vi "PDF_Interface_PDF Protokoll O2 Leaktest.vi"(8 "error in (no error)":errorcluster caption="Fehler (Eingang, kein Fehler)", 11 "Save PDF File Path":path) -> (0 "error out":errorcluster caption="Fehler (Ausgang)")   [LabVIEW 2020, in "O2 Dichtheitstest.lvlib"]
uses:
  O2 Dichtheitstest.lvlib
  Sprachverwaltung/FGV Aktion Tabelle zerlegen.ctl
  Seiten/System Einstellungen V2/Aktioen FGV System Konstanten.ctl
  Aktion FGV O2 Leak.ctl
  PDF_Interface/PDF Protokoll Standard Kopf Optionen.ctl
  <vilib>/Simplicity AI/SAI_PDF_API/Classes/Context/Controls/SAI_PDF_PDF Details.ctl
  PDF_Interface/PDF Interface Helper/PDFContentType.ctl
  PDF_Interface/PDF Interface Helper/PDFTableContentType.ctl
  PDF_Interface/PDF Interface Helper/PDFResults.ctl
  PDF_Interface/PDF Interface Helper/PDFResultPictures.ctl
  PDF_Interface/PDF Interface Helper/PDFCommentPosition.ctl
  PDF_Interface/PDF Interface Helper/PDFPageBreak.ctl
  PDF_Interface/PDF Interface Helper/PDFTablePictures.ctl
  PDF_Interface/PDF Interface Helper/PDFBemerkung.ctl
  <vilib>/Simplicity AI/SAI_PDF_API/Classes/Context/Controls/SAI_PDF_Text Align.ctl
  <vilib>/Simplicity AI/SAI_PDF_API/Classes/Context/Controls/SAI_PDF_Font.ctl
  <vilib>/Simplicity AI/SAI_PDF_API/Classes/Context/Controls/SAI_PDF_Font Encoding.ctl
  Allgemein/allgemeine Sub-VIs.lvlib
  Seiten/System Einstellungen V2/System Einstellungen V2.lvlib
  Sprachverwaltung/Sprachverwaltung.lvlib
  PDF_Interface/PDF Interface.lvlib
  <vilib>/Simplicity AI/SAI_PDF_API/Classes/Context/Context.lvclass
  PDF_Interface/PDF Interface Helper/PDF Interface Helper.lvlib
  Linearisierung V2/Protokoll/Protokoll.lvlib
panel:
  out "Grenzwert Messgasdruck:":string
  out "Messgasdruck:":string
  out "Grenzwert O2:":string
  out "Bestanden":bool caption="Boolesch"
  out "Nullgas Messwert:":string
  out "Datenerfassungszeit:":string
  out "Nullgas Aufschaltzeit:":string
  out "Analysator:":string
  out "Aufschaltpunkt:":string
  out "Endzeit:":string
  out "Startzeit:":string
  out "Ser.Nr.:":string caption="Serien Nummer:"
  out "Messgerät:":string
  # "O2 Leaktest"
  # "s"
  # "s"
  # "kPa"
  # "%"
  # "IAG-Industrie Automatisierungsgeschellschaft m.b.H.    l  Industriestraße 2    l    2722Weikersdorf     )+43262221734 7+43262221734655"
  # "kPa"
  # "%"
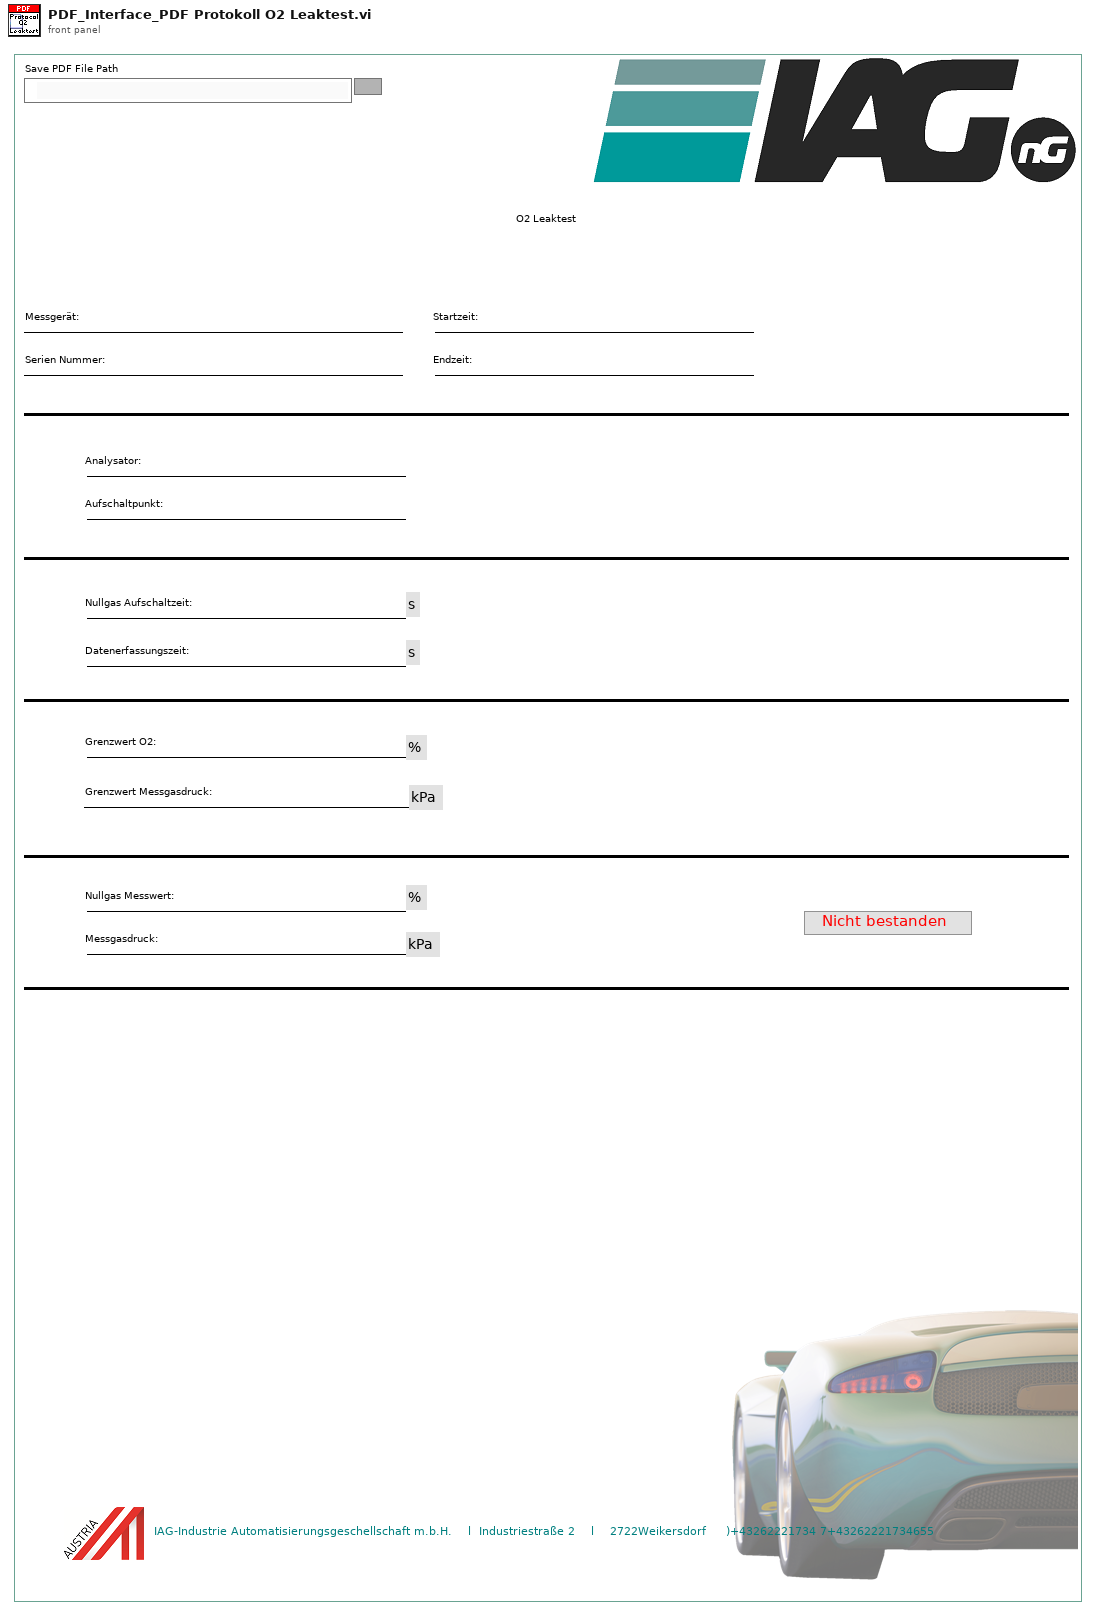
[diagram p1: front panel]
types:
  T1 = typedef "Sprachverwaltung.lvlib/FGV Aktion Tabelle zerlegen.ctl" = enum16{"laden", "vereinzeln", "speichern"}
  T2 = typedef "PDF Interface.lvlib/PDF Protokoll Standard Kopf Optionen.ctl" = cluster{"Analysator":bool, "FT-IR Rezept":bool, "Gasteiler":bool, "Gas Komponente":bool, "Gas Flasche":bool, "LIN Protokoll":bool, "Operator":bool}
  T3 = typedef "O2 Dichtheitstest.lvlib/Aktion FGV O2 Leak.ctl" = enum16{"lesen", "O2 settings", "Pfad", "Protokoll", "laden", "speichern"}
  T4 = typedef "System Einstellungen V2.lvlib/Aktioen FGV System Konstanten.ctl" = enum16{"lesen", "laden", "speichern", "Sprache"}
  T5 = typedef "PDF Interface.lvlib/PDF Interface Helper.lvlib/PDFBemerkung.ctl" = cluster{"Bemerkung Text":string, "Align (Left)":T6, "Add Line Feeds (F:No)":bool, "Font":T7}
  T6 = typedef "SAI_PDF_Toolkit.lvlib/Context.lvclass/SAI_PDF_Text Align.ctl" = i32
  T7 = typedef "SAI_PDF_Toolkit.lvlib/Context.lvclass/SAI_PDF_Font.ctl" = cluster{"Font":string, "Size":i32, "Colour":u32, "Bold":bool, "Italic":bool, "Underline":bool, "Strikethrough":bool, "Font Encoding":T8}
  T8 = typedef "SAI_PDF_Toolkit.lvlib/Context.lvclass/SAI_PDF_Font Encoding.ctl" = enum16{"Cp1252, WinANSI", "IdentityH", "IdentityV", "Cp1250", "Cp1257", "MacRoman"}
  T9 = typedef "PDF Interface.lvlib/PDF Interface Helper.lvlib/PDFResults.ctl" = cluster{"Results":cluster{"Result Text":string, "Result":bool}[], "ResultPictures":T10, "use Pictures":bool, "Image Scale (%)":sgl, "Autoscale? (T)":bool, "Horizontal Align":i32, "Position":i32}
  T10 = typedef "PDF Interface.lvlib/PDF Interface Helper.lvlib/PDFResultPictures.ctl" = cluster{"Yes Ctl Refnum":refnum<vi>, "No Ctl Refnum":refnum<vi>}
  T11 = typedef "PDF Interface.lvlib/PDF Interface Helper.lvlib/PDFTableContentType.ctl" = cluster{"TableHeader":string[], "Table":string[][], "Relative Column Widths (%)":sgl[], "Results":T9, "PositionBemerkung":T12, "PageBreak":T13, "TablePictures":T14, "Horizontal Align":i32}
  T12 = typedef "PDF Interface.lvlib/PDF Interface Helper.lvlib/PDFCommentPosition.ctl" = enum16{"before", "after"}
  T13 = typedef "PDF Interface.lvlib/PDF Interface Helper.lvlib/PDFPageBreak.ctl" = enum16{"none", "before", "after", "after comment"}
  T14 = typedef "PDF Interface.lvlib/PDF Interface Helper.lvlib/PDFTablePictures.ctl" = cluster{"Ctl Refnum In":refnum<vi>[], "RowOrColumn":enum16{"Row", "Column"}, "IndexToInsert":u16, "Image Scale (%)":sgl[], "Autoscale? (T)":bool[], "Horizontal Align":i32}
  T15 = typedef "PDF Interface.lvlib/PDF Interface Helper.lvlib/PDFContentType.ctl" = cluster{"Titel":string, "Header Table":string[][], "Table Array":T11[], "Bemerkungen":T5[]}
  T16 = typedef "SAI_PDF_Toolkit.lvlib/Context.lvclass/SAI_PDF_PDF Details.ctl" = cluster{"Title":string, "Subject":string, "Keywords":string, "Author":string, "Creator":string}
  T17 = cluster{"Header Footer Text Cluster":cluster{"Header Text":string, "Footer Text":string, "Time":string, "Page Number":string}, "PDF Details":T16}
  T18 = typedef "O2 Dichtheitstest.lvlib/O2 Settings.ctl" = cluster{"Kalibriergas":T19, "Aufschaltpunkt":T19, "Nullgas Aufschaltzeit:":sgl, "Datenerfassungszeit:":sgl, "Grenzwert: O2":sgl, "Grenzwert: Messgasdruck":sgl, "Grenzwert: Messgasdruck 2":sgl}
  T19 = typedef "Auswahlfeld.ctl" = u16
  T20 = typedef "O2 Dichtheitstest.lvlib/Protokoll LeakTest.ctl" = cluster{"O2":sgl, "Messgasdruck":sgl, "Startzeit":timestamp, "Endzeit":timestamp, "Bestanden?":bool}
  T21 = cluster{"Header Size":i32, "Column Ratio left":sgl[]}
  T22 = typedef "String - Ausgabefeld.ctl" = string
  T23 = cluster{"Modell":string, "ProjektNummer":string, "Software Version":string, "Seriennummer":string}
  T24 = cluster{"String - Ausgabefeld":T22, "Bestanden?":bool}
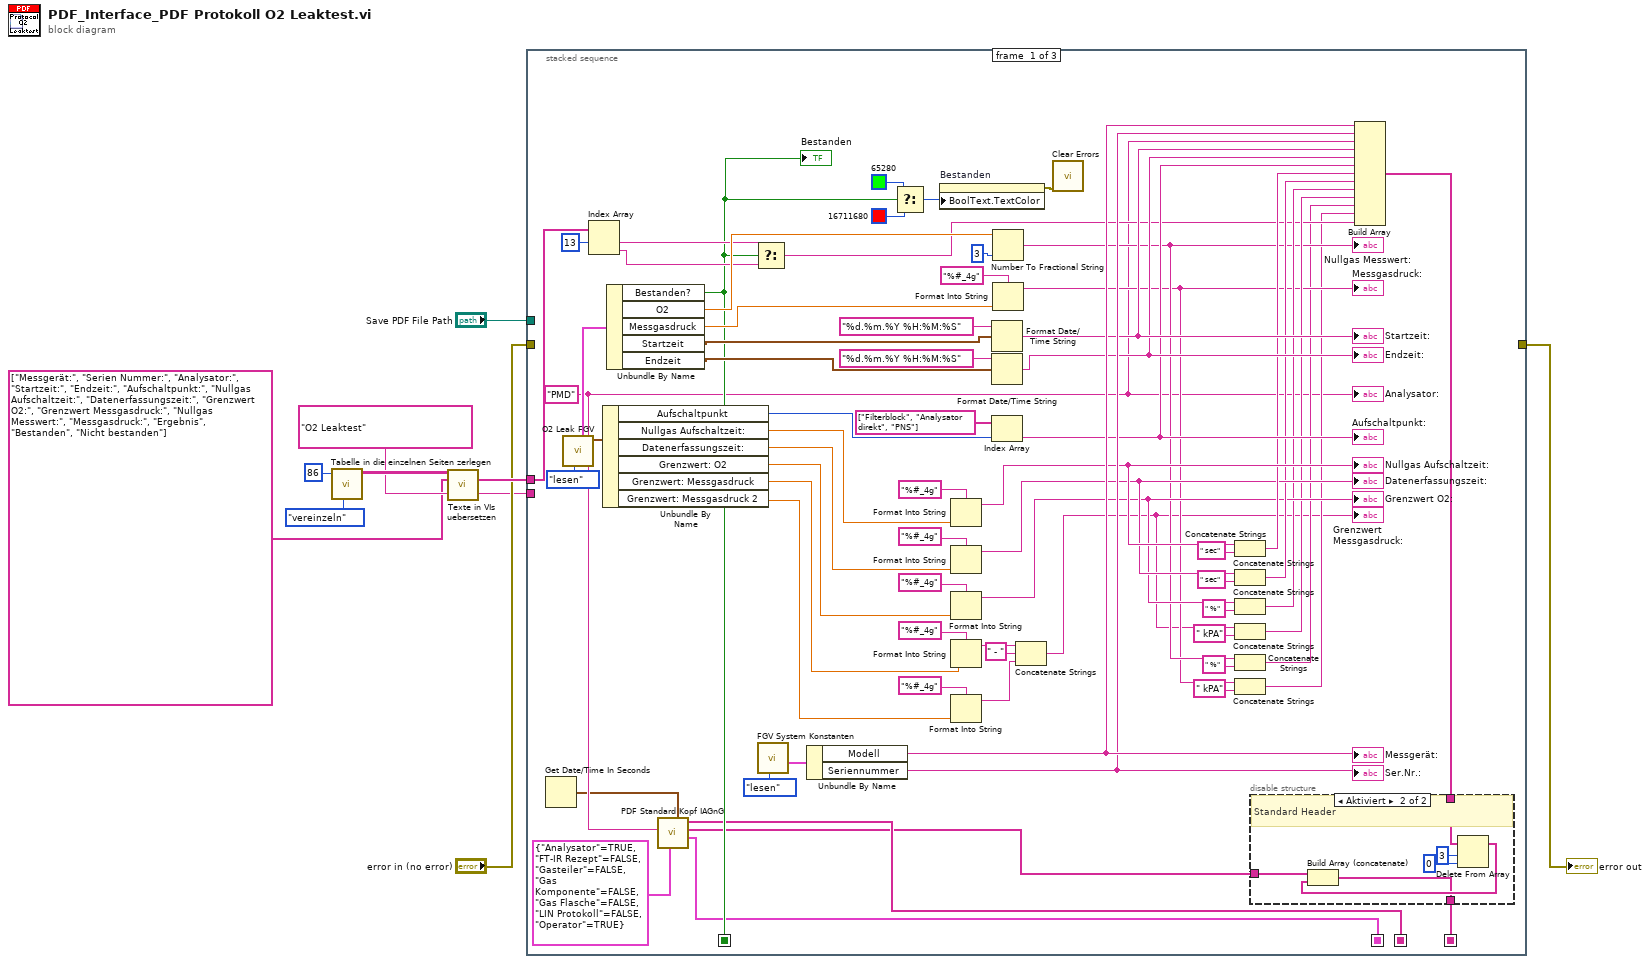
[diagram p0: block diagram]
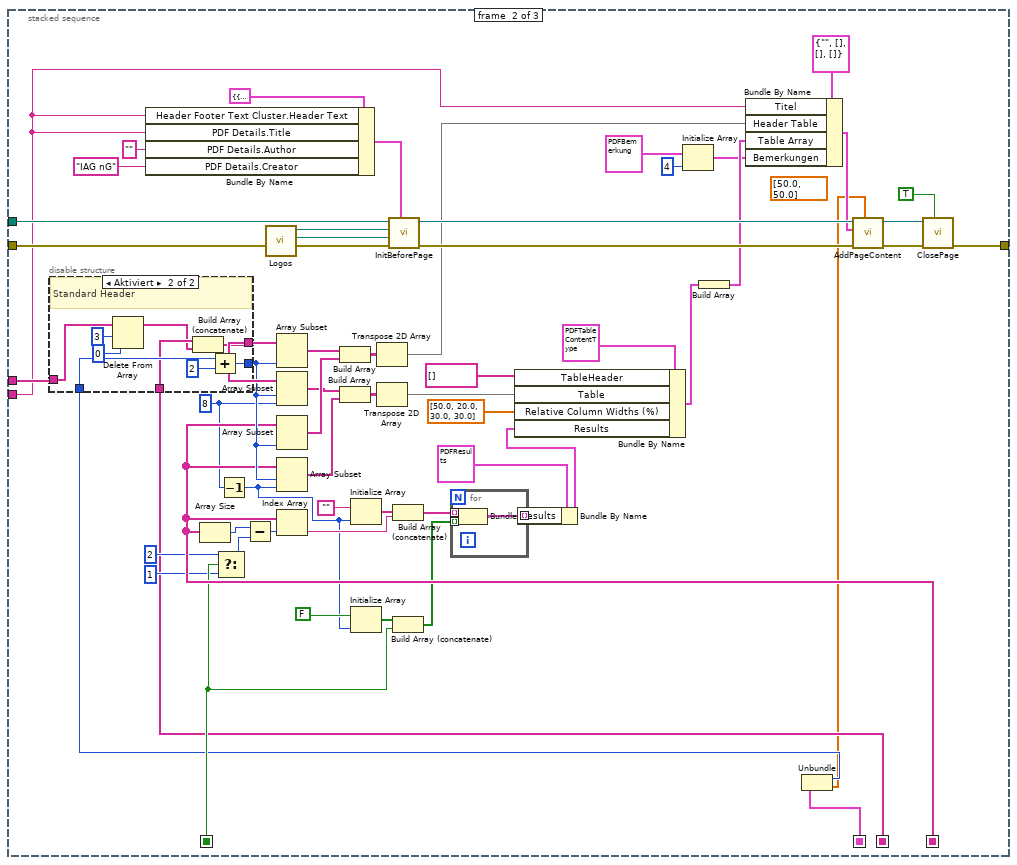
[diagram p3: hidden frame]
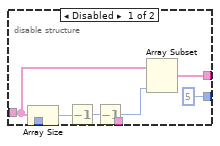
[diagram p4: hidden frame]
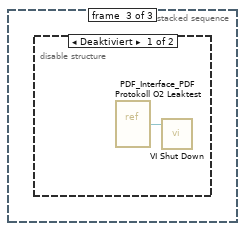
[diagram p5: hidden frame]
diagram:
  n1 = call "Tabelle in die einzelnen Seiten zerlegen.vi"("Aktion"=FGV_Aktion_Tabelle_zerlegen."vereinzeln", "Index (Seite)"=86) -> ("Sprachliste"=w8:string[][])  [unwired: 7 in, 2 out]
  n2 = call "Texte in VIs uebersetzen.vi"("Sprachliste"=w8, "String-Array zum Übersetzen"=string[] ["Messgerät:", "Serien Nummer:", "Analysator:", "Startzeit:", "Endzeit:", "Aufschaltpunkt:", "Nullgas Aufschaltzeit:", "Datenerfassungszeit:", "Grenzwert O2:", "Grenzwert Messgasdruck:", "Nullgas Messwert:", "Messgasdruck:", "Ergebnis", "Bestanden", "Nicht bestanden"], "String zum Übersetzen"="O2 Leaktest") -> ("String-Array zum Übersetzen"=w5:string[], "String zum Übersetzen"=w2:string)  [unwired: 8 in, 3 out]
  n3 = stacked-sequence {
    seq-local: [w16 _ _] -> [_ w124 _]
    seq-local: [w20 _ _] -> [_ w96 _]
    seq-local: [w13 _ _] -> [_ w90 _]
    seq-local: [w14 _ _] -> [_ w89 _]
    tunnel: w5 -> [w42 w137 _]
    tunnel: "error in (no error)" -> [_ w143 _]
    tunnel: "Save PDF File Path" -> [_ w134 _]
    tunnel: w2 -> [_ w130 _]
    tunnel: [_ w107 _] -> w1
    frame #0 {
      w17 = "PMD" ("Analysator:")
      n4 = Get Date/Time In Seconds() -> (seconds since 1Jan1904=w11:timestamp)
      n5 = call "O2 Leak FGV.vi"("Aktion"=Aktion_FGV_O2_Leak."lesen") -> ("O2 Settings"=w62:T18, "Protokoll"=w63:T20)  [unwired: 6 in, 3 out]
      n6 = Index Array(array=w42, index #1=13 ("Index")) -> (element #1=w40:string, element #2=w39:string)  [unwired: 1 in]
      n7 = Unbundle By Name(w62) -> ("Aufschaltpunkt"=w59:T19, "Nullgas Aufschaltzeit:"=w57:sgl, "Datenerfassungszeit:"=w56:sgl, "Grenzwert: O2"=w55:sgl, "Grenzwert: Messgasdruck"=w54:sgl, "Grenzwert: Messgasdruck 2"=w53:sgl)
      n8 = Unbundle By Name(w63) -> ("Bestanden?"=w20:bool, "O2"=w48:sgl, "Messgasdruck"=w58:sgl, "Startzeit"=w61:timestamp, "Endzeit"=w60:timestamp)
      "Bestanden" <- w20
      n9 = call "PDF Standard Kopf IAGnG.vi"("Zeitstempel"=w11, "Oprtionen Cluster"=T2 {"Analysator"=TRUE, "FT-IR Rezept"=FALSE, "Gasteiler"=FALSE, "Gas Komponente"=FALSE, "Gas Flasche"=FALSE, "LIN Protokoll"=FALSE, "Operator"=TRUE}, "Analysator"=w17) -> ("Size Cluster"=w14:T21, "Header Values"=w12:T22[], "Header Labels"=w13:string[])  [unwired: 5 in, 1 out]
      n10 = Select(t=w40, s=w20, f=w39) -> (s? t:f=w25:string)
      n11 = call "FGV System Konstanten.vi"("Aktionen"=Aktioen_FGV_System_Konstanten."lesen") -> ("Cluster out"=w78:T23)  [unwired: 6 in, 4 out]
      n12 = Unbundle By Name(w78) -> ("Modell"=w47:string, "Seriennummer"=w46:string)
      "Messgerät:" <- w47
      "Ser.Nr.:" <- w46
      n13 = Select(t=u32 65280, s=w20, f=u32 16711680) -> (s? t:f=w66:u32)
      n14 = property on="Bestanden" class="Bool. (strikt)"("BoolText.TextColor"=w66) -> (error out=w65:errorcluster)  [unwired: 2 in, 1 out]
      n15 = Format Into String(format string="%#_4g" ("Format-String"), w57) -> (resulting string=w37:string)  [unwired: 2 in, 1 out]
      "Nullgas Aufschaltzeit:" <- w37
      n16 = Format Into String(format string="%#_4g" ("Format-String"), w56) -> (resulting string=w34:string)  [unwired: 2 in, 1 out]
      "Datenerfassungszeit:" <- w34
      n17 = Format Into String(format string="%#_4g" ("Format-String"), w55) -> (resulting string=w28:string)  [unwired: 2 in, 1 out]
      "Grenzwert O2:" <- w28
      n18 = Format Into String(format string="%#_4g" ("Format-String"), w54) -> (resulting string=w70:string)  [unwired: 2 in, 1 out]
      n19 = Format Into String(format string="%#_4g" ("Format-String"), w53) -> (resulting string=w52:string)  [unwired: 2 in, 1 out]
      n20 = Format Date/Time String(time format string (%c)="%d.%m.%Y %H:%M:%S" ("Zeitformatierungs-String (%c)"), seconds (now)=w61) -> (date/time string=w45:string)  [unwired: 1 in]
      "Startzeit:" <- w45
      n21 = Format Date/Time String(time format string (%c)="%d.%m.%Y %H:%M:%S" ("Zeitformatierungs-String (%c)"), seconds (now)=w60) -> (date/time string=w44:string)  [unwired: 1 in]
      "Endzeit:" <- w44
      n22 = Index Array(array=string[] ["Filterblock", "Analysator direkt", "PNS"], index=w59) -> (element=w43:string)
      "Aufschaltpunkt:" <- w43
      n23 = Number To Fractional String(number=w48, precision (6)=i16 3 ("Breite (-)")) -> (F-format string=w24:string)  [unwired: 2 in]
      "Nullgas Messwert:" <- w24
      n24 = Format Into String(format string="%#_4g" ("Format-String"), w58) -> (resulting string=w23:string)  [unwired: 2 in, 1 out]
      "Messgasdruck:" <- w23
      n25 = Concatenate Strings(w70, " - " ("String"), w52) -> (w19:string)
      "Grenzwert Messgasdruck:" <- w19
      n26 = call <vilib>:"Clear Errors.vi"("error in (no error)"=w65) -> ()  [unwired: 5 in, 2 out]
      n27 = Concatenate Strings(w37, " sec" ("String")) -> (w36:string)
      n28 = Concatenate Strings(w34, " sec" ("String")) -> (w33:string)
      n29 = Concatenate Strings(w28, " %" ("String")) -> (w27:string)
      n30 = Concatenate Strings(w19, " kPA" ("String")) -> (w26:string)
      n31 = Concatenate Strings(w24, " %" ("String")) -> (w22:string)
      n32 = Concatenate Strings(w23, " kPA" ("String")) -> (w21:string)
      n33 = Build Array(w47, w46, w17, w45, w44, w43, w36, w33, w27, w26, w22, w21, w25) -> (w15:string[])
      n34 = disable-structure shown="Aktiviert" {
        disable-tunnel: [w80 w81] -> w16
        disable-tunnel: w15 -> [w80 w85]
        disable-tunnel: w12 -> [_ w86]
        frame Disabled {
        }
        frame Enabled {
          # "Standard Header"
          n35 = Delete From Array(array=w85, length=3 ("Länge"), index=0 ("Index")) -> (array with subset deleted=w82:string[])  [unwired: 1 out]
          n36 = Build Array (concatenate)(w86, w82) -> (w81:T22[])
        }
      }
      "Analysator:" <- w17
    }
    frame #1 {
      (unwired) sgl[] [50.0, 50.0] ("Column Ratio left")
      w92 = 8 ("Länge")
      n37 = Bundle By Name(cluster=T17 {"Header Footer Text Cluster"={"Header Text"="Protokoll XYZ", "Footer Text"="IAG nG", "Time"="<TIMESTAMP yyyy-MM-dd>", "Page Number"="Page <P> of <PT>"}, "PDF Details"={"Title"="Test PDF", "Subject"="Versa Tabasco", "Keywords"="", "Author"="RIW", "Creator"="IAG"}} ("Info"), "Header Footer Text Cluster.Header Text"=w130, "PDF Details.Title"=w130, "PDF Details.Author"="", "PDF Details.Creator"="IAG nG") -> (w132:T17)
      n38 = Array Size(array=w124) -> (size(s)=w123:i32)
      n39 = Select(t=2 ("Länge"), s=w96, f=1 ("Länge")) -> (s? t:f=w95:i32)
      n40 = Decrement(x=w92) -> (x-1=w91:i32)
      n41 = Subtract(x=w123, y=w95) -> (x-y=w115:i32)
      n42 = call "Logos.vi"() -> ("Footer Image File Path"=w144:path, "Header Image File Path"=w145:path)  [unwired: 8 in, 2 out]
      n43 = Index Array(array=w124, index=w115) -> (element=w120:T22)
      n44 = Initialize Array("", w91) -> (w121:string[])
      n45 = Initialize Array(FALSE, w91) -> (w113:bool[])
      n46 = call "InitBeforePage.vi"("Info"=w132, "Fehler (Eingang, kein Fehler)"=w143, "Footer Image File Path"=w144, "Header Image File Path"=w145, "Path (Dialog if Empty)"=w134) -> ("Fehler (Ausgang)"=w142:errorcluster, "Context (Ausgang)"=w141:refnum<class "Context.lvclass">)  [unwired: 5 in]
      n47 = Build Array (concatenate)(w121, w120) -> (w112:T22[])
      n48 = Build Array (concatenate)(w113, w96) -> (w111:bool[])
      n49 = for {
        tunnel: w112 -> [w163] mode=indexing
        tunnel: w111 -> [w162] mode=indexing
        tunnel: [w161] -> w98 mode=indexing
        n50 = Bundle("String - Ausgabefeld"=w163, "Bestanden?"=w162) -> (w161:T24)  [unwired: 1 in]
      }
      n51 = Bundle By Name(cluster=T9 {"Results"=[], "ResultPictures"={"Yes Ctl Refnum"=refnum, "No Ctl Refnum"=refnum}, "use Pictures"=FALSE, "Image Scale (%)"=100.0, "Autoscale? (T)"=TRUE, "Horizontal Align"=3, "Position"=0} ("Results"), "Results"=w98) -> (w99:T9)
      n52 = Initialize Array(T5 {"Bemerkung Text"="", "Align (Left)"=0, "Add Line Feeds (F:No)"=FALSE, "Font"={"Font"="Arial", "Size"=10, "Colour"=0, "Bold"=FALSE, "Italic"=FALSE, "Underline"=FALSE, "Strikethrough"=FALSE, "Font Encoding"=enum."Cp1252, WinANSI"}} ("Bemerkung"), 4 ("Dimensionsgröße")) -> (w102:T5[])
      n53 = Unbundle(w89) -> ("Header Size"=w88:i32, "Column Ratio left"=w87:sgl[])
      n54 = disable-structure shown="Aktiviert" {
        disable-tunnel: w137 -> [w148 w157]
        disable-tunnel: [w147 w153] -> w126
        disable-tunnel: [5 ("Länge") w159] -> w125
        disable-tunnel: w90 -> [_ w154]
        disable-tunnel: w88 -> [_ w160]
        frame Disabled {
          n55 = Array Size(array=w148) -> (size(s)=w151:i32)
          n56 = Decrement(x=w151) -> (x-1=w150:i32)
          n57 = Decrement(x=w150) -> (x-1=w149:i32)
          n58 = Array Subset(array=w148, length=w149) -> (w147:string[])  [unwired: 1 in]
        }
        frame Enabled {
          # "Standard Header"
          n59 = Delete From Array(array=w157, length=3 ("Länge"), index=0 ("Index")) -> (array with subset deleted=w152:string[])  [unwired: 1 out]
          n60 = Build Array (concatenate)(w154, w152) -> (w153:string[])
          n61 = Add(x=w160, y=2) -> (x+y=w159:i32)
        }
      }
      n62 = Array Subset(array=w126, length=w125) -> (w129:string[])  [unwired: 1 in]
      n63 = Array Subset(array=w126, index=w125, length=w92) -> (w118:string[])
      n64 = Array Subset(array=w124, length=w125) -> (w128:T22[])  [unwired: 1 in]
      n65 = Array Subset(array=w124, index=w125, length=w91) -> (w117:T22[])
      n66 = Build Array(w129, w128) -> (w127:T22[][])
      n67 = Build Array(w118, w117) -> (w116:T22[][])
      n68 = Transpose 2D Array(2D array=w127) -> (transposed array=w105:T22[][])
      n69 = Transpose 2D Array(2D array=w116) -> (transposed array=w104:T22[][])
      n70 = Bundle By Name(cluster=T11 {"TableHeader"=[], "Table"=[], "Relative Column Widths (%)"=[], "Results"={"Results"=[], "ResultPictures"={"Yes Ctl Refnum"=refnum, "No Ctl Refnum"=refnum}, "use Pictures"=FALSE, "Image Scale (%)"=0.0, "Autoscale? (T)"=FALSE, "Horizontal Align"=0, "Position"=0}, "PositionBemerkung"=enum."before", "PageBreak"=enum."none", "TablePictures"={"Ctl Refnum In"=[], "RowOrColumn"=enum."Row", "IndexToInsert"=0, "Image Scale (%)"=[], "Autoscale? (T)"=[], "Horizontal Align"=0}, "Horizontal Align"=0} ("Table Array"), "TableHeader"=string[] [], "Table"=w104, "Relative Column Widths (%)"=sgl[] [50.0, 20.0, 30.0, 30.0], "Results"=w99) -> (w109:T11)
      n71 = Build Array(w109) -> (w108:T11[])
      n72 = Bundle By Name(cluster=T15 {"Titel"="", "Header Table"=[], "Table Array"=[], "Bemerkungen"=[]} ("Content"), "Titel"=w130, "Header Table"=w105, "Table Array"=w108, "Bemerkungen"=w102) -> (w106:T15)
      n73 = call "AddPageContent.vi"("Column Ratio left"=w87, "error in"=w142, "Content"=w106, "Context (Eingang)"=w141) -> ("error out"=w140:errorcluster, "Context (Ausgang)"=w139:refnum<class "Context.lvclass">)  [unwired: 6 in]
      n74 = call "ClosePage.vi"("popup viewer"=TRUE, "Fehler (Eingang, kein Fehler)"=w140, "Context (Eingang)"=w139) -> ("Fehler (Ausgang)"=w107:errorcluster)  [unwired: 8 in]
    }
    frame #2 {
      n75 = disable-structure shown="Deaktiviert" {
        frame Disabled {
          n76 = vi-ref "PDF_Interface_PDF Protokoll O2 Leaktest.vi"() -> (w164:refnum<vi>)
          n77 = call "VI Shut Down.vi"("VI Referenz"=w164) -> ()  [unwired: 11 in]
        }
        frame Enabled {
        }
      }
    }
  }
  "error out" <- w1
